vi "Write Size.vi"(5 "Size":T1, 9 "IOName in":refnum<class "IOName.lvclass">) -> (3 "IOName out":refnum<class "IOName.lvclass">)   [LabVIEW 2014, in "Raspberry Pi Compatible Compiler for LabVIEW.lvlib" / "IOName.lvclass"]
uses:
  IOName.lvclass
  <vilib>/Utility/miscctls.llb/LVBoundsTypeDef.ctl
  IOName.lvclass/IOName.ctl
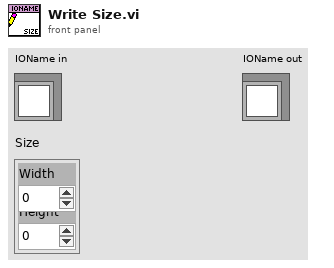
[diagram p1: front panel]
types:
  T1 = typedef "LVBoundsTypeDef.ctl" = cluster{"Width":u32, "Height":u32}
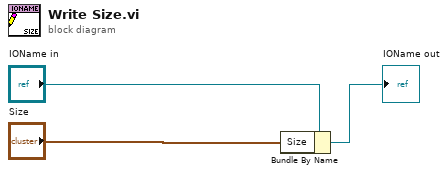
[diagram p0: block diagram]
diagram:
  n1 = Bundle By Name(cluster="IOName in", "Size"="Size") -> (→"IOName out":refnum<class "IOName.lvclass">)
